vi "파일.vi"() -> ()   [LabVIEW 2014]
panel:
  in  "error in (no error)":errorcluster
  out "error out":errorcluster
  out "경로 배열":path[](array[path])
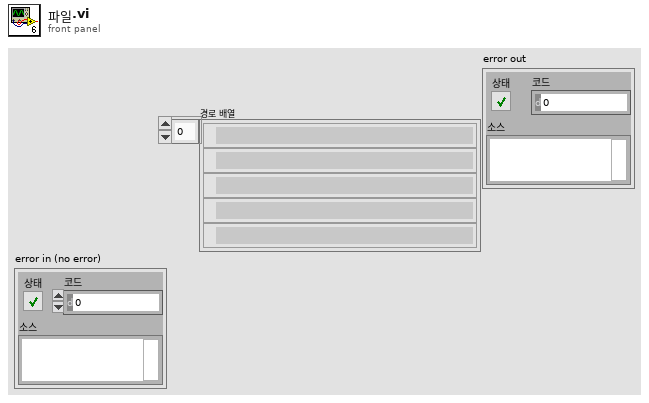
[diagram p1: front panel]
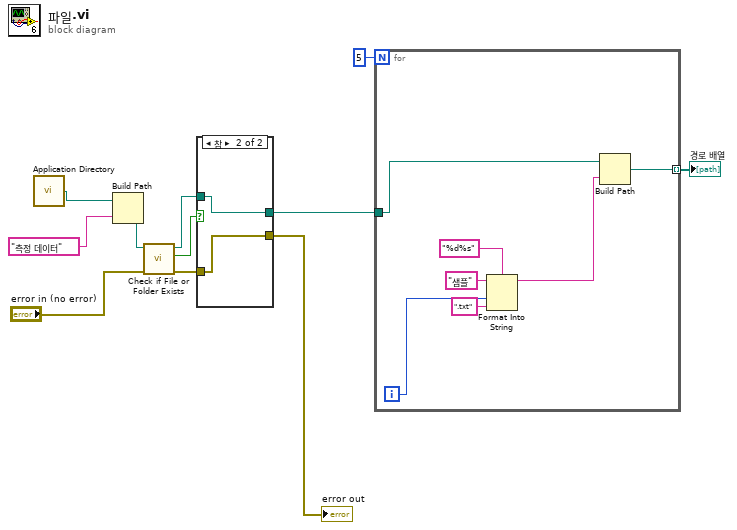
[diagram p0: block diagram]
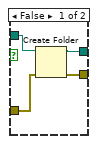
[diagram p2: hidden frame]
diagram:
  n1 = call <vilib>:"Application Directory.vi"() -> ("Application Directory"=w10:path)
  n2 = Build Path(base path=w10, name or relative path="측정 데이터" ("이름 또는 상대 경로")) -> (appended path=w5:path)
  n3 = call <vilib>:"Check if File or Folder Exists.vi"("error in (no error)"="error in (no error)", "path"=w5) -> ("error out"=w2:errorcluster, "file or folder exists?"=w1:bool, "dup path"=w3:path)  [unwired: 7 in]
  n4 = case shown="참" w1 {
    tunnel: [w15 w17] -> w7
    tunnel: [w14 w16] -> w6
    tunnel: w3 -> [w13 w17]
    tunnel: w2 -> [w12 w16]
    frame False {
      n5 = Create Folder(path (use dialog)=w13, error in=w12) -> (created path=w15:path, error out=w14:errorcluster)  [unwired: 1 in, 1 out]
    }
    frame True {
    }
  }
  "error out" <- w6
  n6 = for {
    N: 5 -> [_]
    tunnel: w7 -> [w19]
    tunnel: [w18] -> w8 mode=indexing
    i -> [w24]
    n7 = Format Into String(format string="%d%s" ("포맷 문자열"), initial string="샘플" ("초기 문자열"), w24, ".txt" ("입력 2")) -> (resulting string=w20:string)  [unwired: 1 in, 1 out]
    n8 = Build Path(base path=w19, name or relative path=w20) -> (appended path=w18:path)
  }
  "경로 배열" <- w8
